vi "PreliminaryOperations.vi"(8 "error IN":errorcluster, 9 "MainRobotREF_IN":refnum<k24>, 10 "Applications":refnum<k24>, 11 "ClientREF_IN":refnum<k24>) -> (0 "error OUT":errorcluster, 1 "MainRobotREF_OUT":refnum<k24>, 2 "Applications out":refnum<k24>, 3 "ClientREF_OUT":refnum<k24>)   [LabVIEW 2018]
uses:
  C:/GIT/gaialabviewclient/Gaia_LabVIEW/Resources/JOT.GaiaClient.dll
  Gaia_LabVIEW/Resources/JOT.GaiaClient.dll
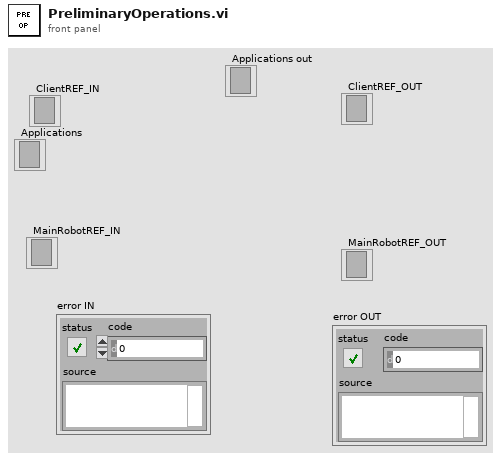
[diagram p1: front panel]
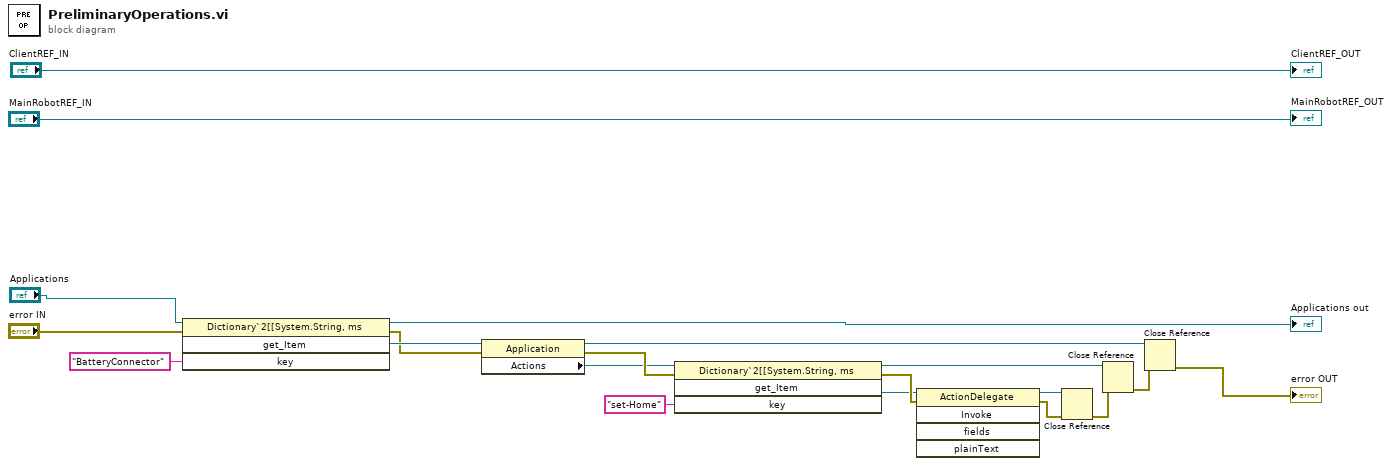
[diagram p0: block diagram]
diagram:
  n1 = invoke class="Dictionary`2[[System.String, ms" method="get_Item"(reference="Applications", error in="error IN", "key"="BatteryConnector") -> (reference out=→"Applications out":refnum<k24>, error out=w11:errorcluster, "get_Item"=w14:refnum<k24>)  [unwired: 1 in, 1 out]
  n2 = property class="Application"(reference=w14, error in=w11) -> (reference out=w7:refnum<k24>, error out=w15:errorcluster, "Actions"=w12:refnum<k24>)
  n3 = invoke class="Dictionary`2[[System.String, ms" method="get_Item"(reference=w12, error in=w15, "key"="set-Home") -> (reference out=w18:refnum<k24>, error out=w16:errorcluster, "get_Item"=w13:refnum<k24>)  [unwired: 1 in, 1 out]
  n4 = invoke class="ActionDelegate" method="Invoke"(reference=w13, error in=w16) -> (reference out=w10:refnum<k24>, error out=w17:errorcluster)  [unwired: 3 in, 3 out]
  n5 = Close Reference(reference=w10, error in (no error)=w17) -> (error out=w9:errorcluster)
  n6 = Close Reference(reference=w18, error in (no error)=w9) -> (error out=w8:errorcluster)
  n7 = Close Reference(reference=w7, error in (no error)=w8) -> (error out=→"error OUT":errorcluster)
  "ClientREF_OUT" <- "ClientREF_IN"
  "MainRobotREF_OUT" <- "MainRobotREF_IN"
